vi "onProcessStarted.vi"(8 "error in (no error)":errorcluster, 11 "MAUI":refnum<class "MAUI.lvclass">) -> (0 "error out":errorcluster, 3 "MAUI out":refnum<class "MAUI.lvclass">)   [LabVIEW 2016, in "MAUI.lvclass"]
doc: "JKI State Machine Objects (SMO) 1.3.0.56\nJKI - JKI\nCopyright (c) 2017, JKI"
uses:
  MAUI.lvclass
  <vilib>/Levylab/Embedded SMO UI/EmbeddedSMO.lvclass
  C:/Program Files (x86)/National Instruments/LabVIEW 2016/vi.lib/JKI/JKI SMO/SMO/SMO.lvclass
  <vilib>/JKI/JKI SMO/SMO.UI/SMO.UI.lvclass
  <vilib>/JKI/JKI SMO/SMO/SMO.lvclass
panel:
  # "For instructions on how to use the JKI State Machine Objects, examples and video tutorials, visit:\nhttp://jki.net/state-machine-objects/\n\nJKI State Machine Objects™\nhttp://jki.net/state-machine-objects/\nCopyright (C) 2005-2015, JKI <info@jki.net>\nALL RIGHTS RESERVED"
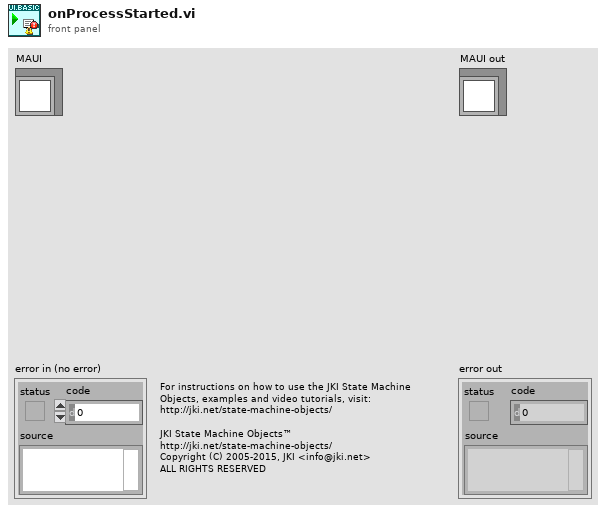
[diagram p1: front panel]
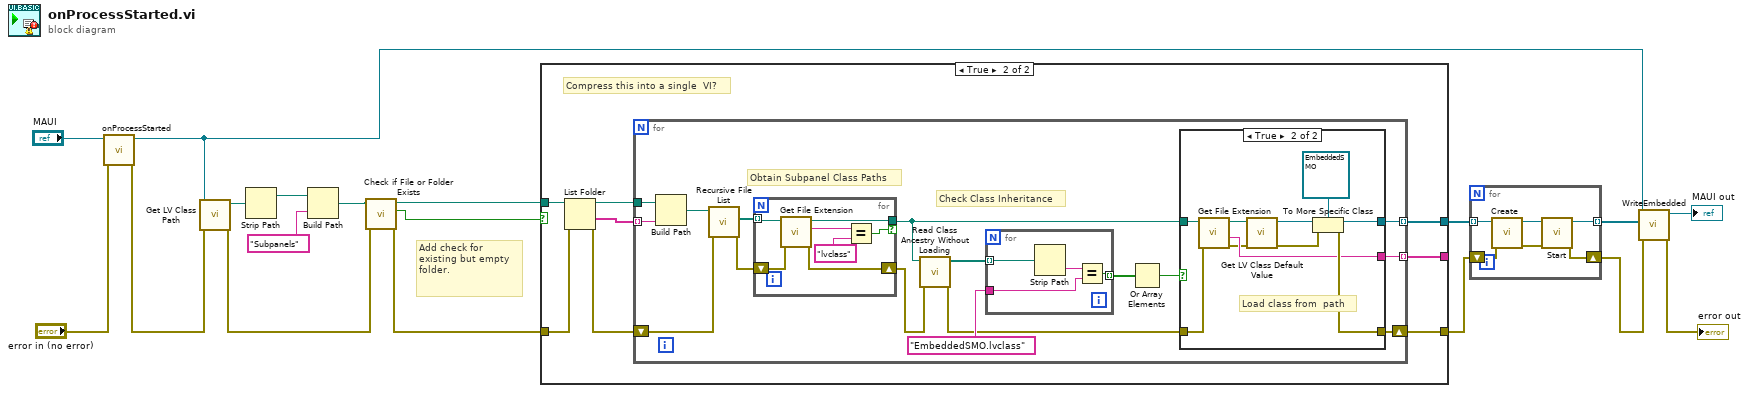
[diagram p0: block diagram]
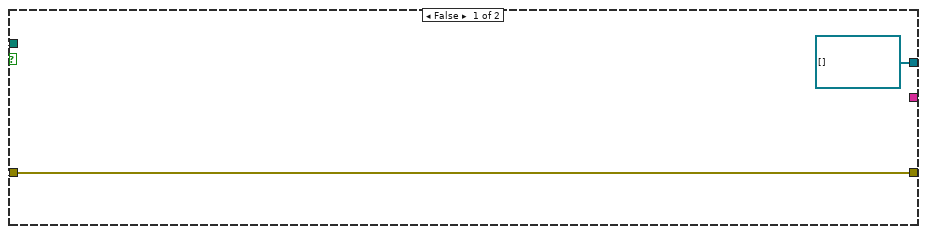
[diagram p2: hidden frame]
diagram:
  # "Add check for existing but empty folder."
  n1 = call-parent "onProcessStarted.vi"("error in (no error)"="error in (no error)", "SMO"="MAUI") -> ("error out"=w8:errorcluster, "SMO out"=w7:refnum<class "MAUI.lvclass">)  [unwired: 8 in]
  n2 = call <vilib>:"Get LV Class Path.vi"("error in (no error)"=w8, "object"=w7) -> ("error out"=w9:errorcluster, "class path"=w16:path)  [unwired: 8 in]
  n3 = Strip Path(path=w16) -> (stripped path=w15:path)  [unwired: 1 out]
  n4 = Build Path(base path=w15, name or relative path="Subpanels") -> (appended path=w13:path)
  n5 = call <vilib>:"Check if File or Folder Exists.vi"("error in (no error)"=w9, "path"=w13) -> ("error out"=w11:errorcluster, "file or folder exists?"=w10:bool, "dup path"=w12:path)  [unwired: 7 in]
  n6 = case shown="True" w10 {
    tunnel: w12 -> [w21 w29]
    tunnel: w11 -> [w20 w24]
    tunnel: [w20 w23] -> w1
    tunnel: [refnum<class "EmbeddedSMO.lvclass">[] [] w25] -> w4
    tunnel: [_ w22] -> _
    frame False {
      n7 = Create Folder(path (use dialog)=w21, error in=w20) -> ()  [unwired: 1 in, 3 out]
    }
    frame True {
      # "Compress this into a single  VI?"
      n8 = List Folder(path=w29, error in=w24) -> (path out=w28:path, folder names=w27:string[], error out=w26:errorcluster)  [unwired: 2 in, 1 out]
      n9 = for {
        tunnel: w28 -> [w45]
        tunnel: w27 -> [w44] mode=indexing
        tunnel: [w40] -> w25 mode=indexing
        shift-right: [w32] -> w23
        shift-left: w26 -> [w36]
        tunnel: [w30] -> w22 mode=indexing
        # "Check Class Inheritance"
        # "Obtain Subpanel Class Paths"
        n10 = Build Path(base path=w45, name or relative path=w44) -> (appended path=w43:path)
        n11 = call <vilib>:"Recursive File List.vi"("error in (no error)"=w36, "Folder Path"=w43) -> ("error out"=w35:errorcluster, "All Files in Dir"=w42:path[])  [unwired: 5 in, 3 out]
        n12 = for {
          tunnel: w42 -> [w65] mode=indexing
          tunnel: [w64] -> w41 if=w63
          shift-right: [w61] -> w34
          shift-left: w35 -> [w62]
          n13 = call <vilib>:"Get File Extension.vi"("error in (no error)"=w62, "file"=w65) -> ("error out"=w61:errorcluster, "lowercase file extension"=w67:string, "dup file"=w64:path)  [unwired: 5 in, 2 out]
          n14 = Equal?(x=w67, y="lvclass") -> (x = y?=w63:bool)
        }
        n15 = call <vilib>:"Read Class Ancestry Without Loading.vi"("error in (no error)"=w34, "LabVIEW Class Path"=w41) -> ("error out"=w33:errorcluster, "Class Ancestry"=w39:path[])  [unwired: 8 in]
        n16 = for {
          tunnel: w39 -> [w60] mode=indexing
          tunnel: [w58] -> w38 mode=indexing
          tunnel: "EmbeddedSMO.lvclass" -> [w57]
          n17 = Strip Path(path=w60) -> (name=w59:string)  [unwired: 1 out]
          n18 = Equal?(x=w59, y=w57) -> (x = y?=w58:bool)
        }
        n19 = Or Array Elements(Boolean array=w38) -> (logical OR=w31:bool)
        n20 = case shown="True" w31 {
          tunnel: w41 -> [_ w51]
          tunnel: [_ w56] -> w40
          tunnel: w33 -> [w46 w48]
          tunnel: [w46 w52] -> w32
          tunnel: [_ w49] -> w30
          frame False {
          }
          frame True {
            # "Load class from  path"
            n21 = call <vilib>:"Get File Extension.vi"("error in (no error)"=w48, "file"=w51) -> ("error out"=w47:errorcluster, "filename without extension"=w49:string, "dup file"=w50:path)  [unwired: 5 in, 2 out]
            n22 = call <vilib>:"Get LV Class Default Value.vi"("error in (no error)"=w47, "class path"=w50) -> ("error out"=w53:errorcluster, "object"=w55:refnum<class>)  [unwired: 8 in]
            n23 = To More Specific Class(target class=refnum<class "EmbeddedSMO.lvclass"> refnum ("EmbeddedSMO"), reference=w55, error in=w53) -> (specific class reference=w56:refnum<class "EmbeddedSMO.lvclass">, error out=w52:errorcluster)
          }
        }
      }
    }
  }
  n24 = for {
    tunnel: w4 -> [w73] mode=indexing
    tunnel: [w72] -> w3 mode=indexing
    shift-right: [w68] -> w2
    shift-left: w1 -> [w69]
    n25 = call <vilib>:"Create.vi"("error in (no error)"=w69, "SMO"=w73) -> ("error out"=w70:errorcluster, "SMO out"=w71:refnum<class "EmbeddedSMO.lvclass">)  [unwired: 7 in, 1 out]
    n26 = call <vilib>:"Start.vi"("error in (no error)"=w70, "SMO"=w71) -> ("error out"=w68:errorcluster, "SMO out"=w72:refnum<class "EmbeddedSMO.lvclass">)  [unwired: 8 in]
  }
  n27 = call "WriteEmbedded.vi"("error in (no error)"=w2, "Subpanels"=w3, "MAUI in"=w7) -> ("error out"=→"error out":errorcluster, "MAUI out"=→"MAUI out":refnum<class "MAUI.lvclass">)  [unwired: 7 in]
